vi "GT Arc XYZ.vi"(0 "cardNum":i16, 1 "crd":i16, 2 "x":i32, 3 "y":i32, 4 "z":i32, 5 "interX":dbl, 6 "interY":dbl, 7 "error in (no error)":errorcluster caption="错误输入（无错误）", 8 "interZ":dbl, 9 "synVel":dbl, 10 "synAcc":dbl, 11 "velEnd":dbl, 12 "fifo":i16) -> (20 "function return":i16, 27 "error out":errorcluster caption="错误输出")   [LabVIEW 2020, in "gts.lvlib"]
doc: "GT_API GT_ArcXYZ(short cardNum,short crd,long x,long y,long z,double interX,double interY,double interZ,double synVel,double synAcc,double velEnd=0,short fifo=0);"
uses:
  gts.lvlib
  dll/32bit/multi_card/gts.dll
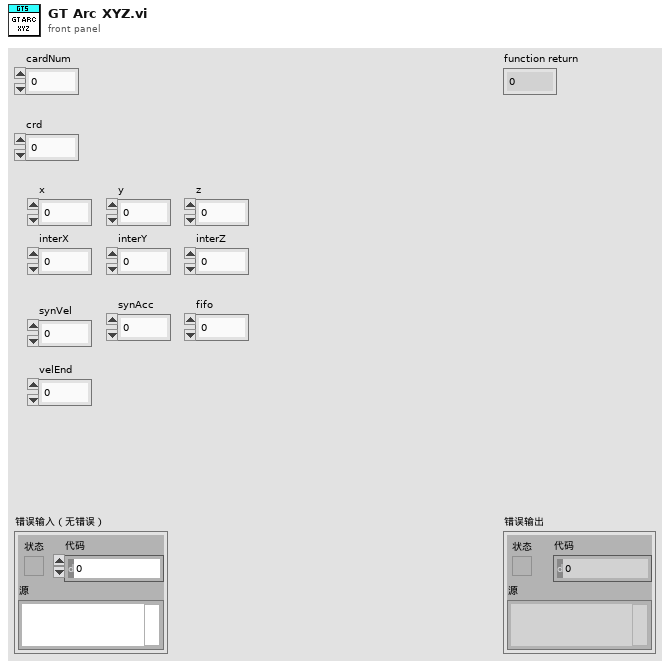
[diagram p1: front panel]
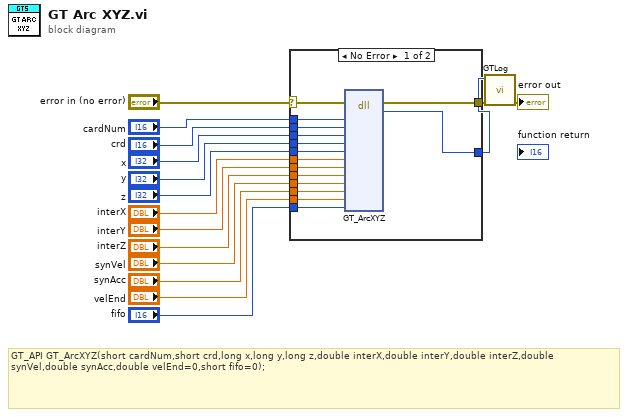
[diagram p0: block diagram]
diagram:
  # "GT_API GT_ArcXYZ(short cardNum,short crd,long x,long y,long z,double interX,double interY,double interZ,double synVel,double synAcc,double velEnd=0,short fifo=0);"
  n1 = case shown="No Error" "error in (no error)" {
    selector: "error in (no error)" -> [w18 w32]
    tunnel: [w31 _] -> w1
    tunnel: "cardNum" -> [w30 _]
    tunnel: "crd" -> [w29 _]
    tunnel: "x" -> [w28 _]
    tunnel: "y" -> [w27 _]
    tunnel: "z" -> [w26 _]
    tunnel: "interX" -> [w25 _]
    tunnel: "interY" -> [w24 _]
    tunnel: "interZ" -> [w23 _]
    tunnel: "synVel" -> [w22 _]
    tunnel: "synAcc" -> [w21 _]
    tunnel: "velEnd" -> [w20 _]
    tunnel: "fifo" -> [w19 _]
    tunnel: [w17 w32] -> w3
    frame No Error {
      n2 = dll-call lib="C:/1228/dll/32bit/multi_card/gts.*" fn="GT_ArcXYZ"(error in=w18, "cardNum"=w30, "crd"=w29, "x"=w28, "y"=w27, "z"=w26, "interX"=w25, "interY"=w24, "interZ"=w23, "synVel"=w22, "synAcc"=w21, "velEnd"=w20, "fifo"=w19) -> (error out=w17:errorcluster, w31:i16)  [unwired: 14 in, 1 out]
    }
    frame Error {
    }
  }
  n3 = call "GTLog.vi"("error in (no error)"=w3, "Numeric"=w1) -> ("error out"=→"error out":errorcluster)  [unwired: 9 in]
